vi "RP Read RX FIFO.vi"(6 "FIFO Bytes per read":i32=49152, 8 "Error In":errorcluster, 11 "connection ID":refnum<k5>) -> (0 "Error Out":errorcluster, 1 "Y":i32[](array[numeric]), 2 "X":i32[](array[numeric]), 3 "connection ID out":refnum<k5>, 4 "F":i32[](array[numeric]))   [LabVIEW 2015]
uses:
  RP Command.ctl
panel:
  out "Waveform Graph":i32[](graph)
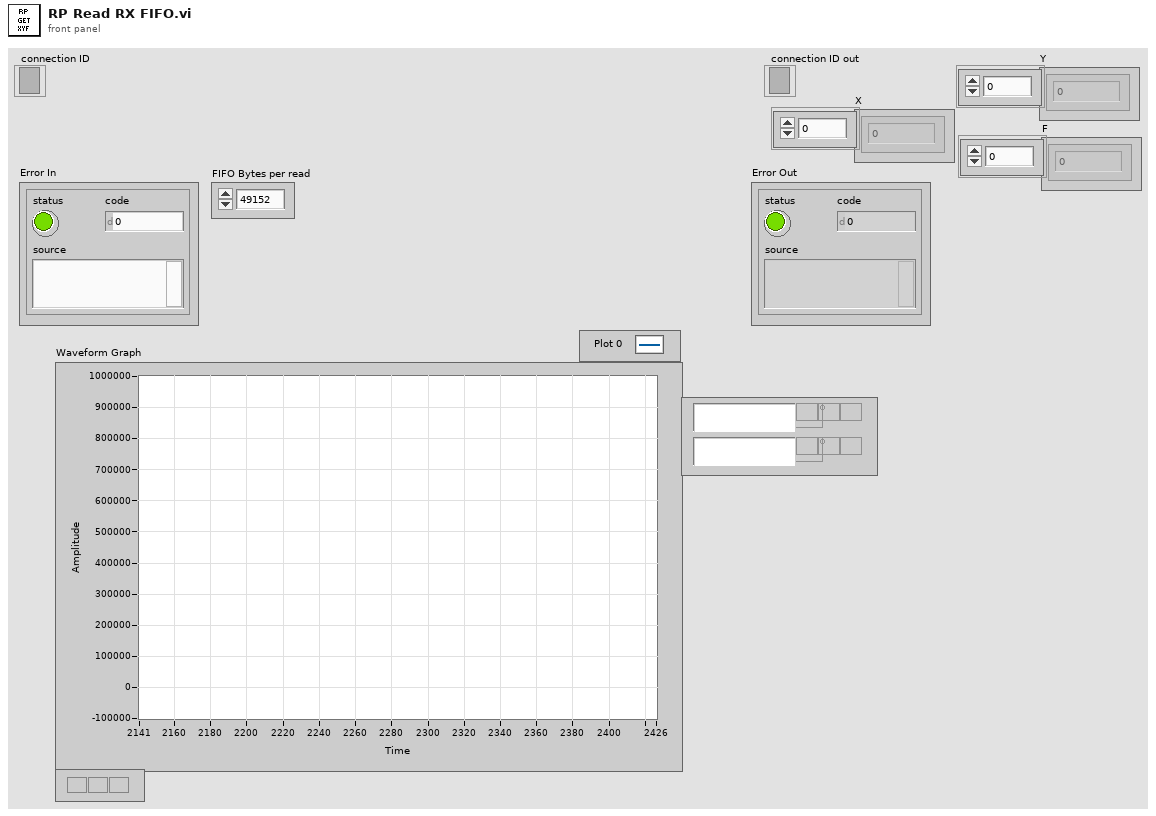
[diagram p1: front panel]
types:
  T1 = typedef "RP Command.ctl" = enum16{"Set frequency", "Read IDN", "Stop server", "Get status", "Get temperature", "Connect client", "Arm", "Software trigger", "Get whole buffer", "Get chunk", "System call", "Get config", "Set config", "Recieve data", "Play pattern", "Transmit data"}
  T2 = enum16{"big-endian, network order", "native, host order", "little-endian"}
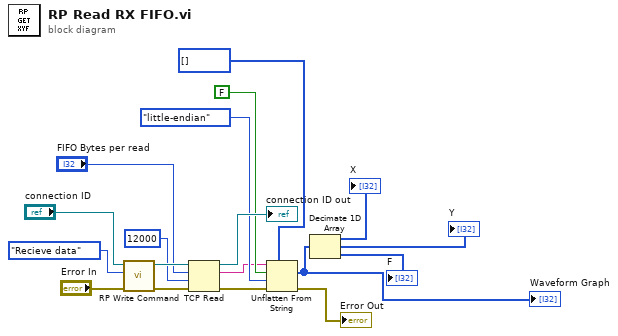
[diagram p0: block diagram]
diagram:
  n1 = call "RP Write Command.vi"("Error In"="Error In", "Command number"=RP_Command."Recieve data", "connection ID"="connection ID") -> ("Error Out"=w17:errorcluster, "connection ID out"=w18:refnum<k5>)  [unwired: 6 in, 1 out]
  n2 = TCP Read(connection ID=w18, bytes to read="FIFO Bytes per read", error in (no error)=w17, 9:12000 ("timeout ms (25000)")) -> (connection ID out=→"connection ID out":refnum<k5>, data out=w8:string, error out=w7:errorcluster)  [unwired: 1 in]
  n3 = Unflatten From String(type=i32[] [], binary string=w8, data includes array or string size? (T)=FALSE, byte order (0:big-endian, network order)=T2."little-endian", error in (no error)=w7) -> (value=w2:i32[], error out=→"Error Out":errorcluster)  [unwired: 1 out]
  "Waveform Graph" <- w2
  n4 = Decimate 1D Array(w2) -> (→"X":i32[], →"Y":i32[], →"F":i32[])
